vi "Configure Bitfile.vi"(0 "USRP RIO device":T1, 5 "which bitfile":string(combo)="Time", 11 "error in":errorcluster) -> (4 "USRP RIO device":T1, 6 "bitfile":path, 15 "error out":errorcluster)   [LabVIEW 2016]
uses:
  <vilib>/userdefined/Silver/nirio_resource_slv.ctl
  <vilib>/Utility/error.llb/Error Cluster From Error Code.vi
  <vilib>/ErrorRing/Error Ring.xnode
  <vilib>/regexp/Match Regular Expression.xnode
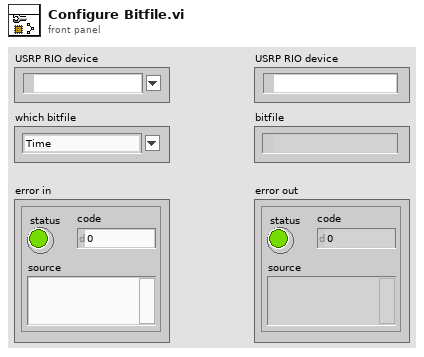
[diagram p1: front panel]
types:
  T1 = typedef "nirio_resource_slv.ctl" = tag
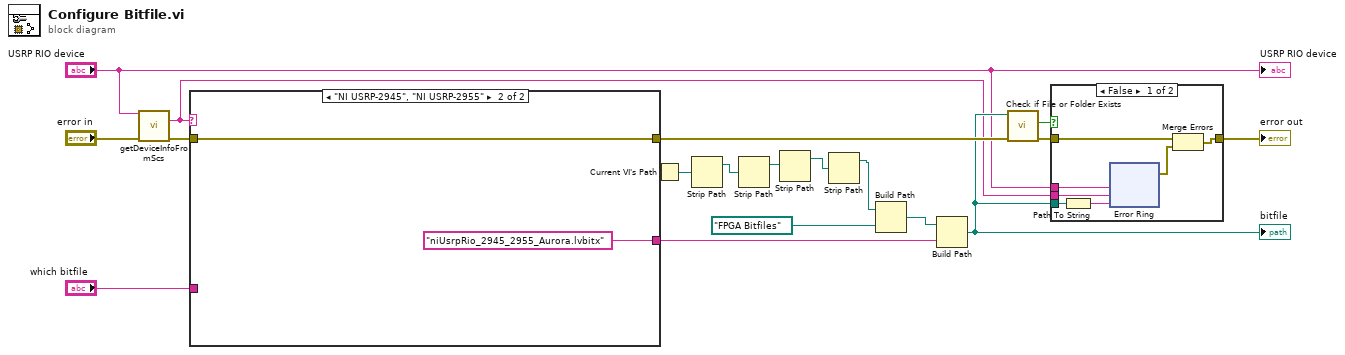
[diagram p0: block diagram]
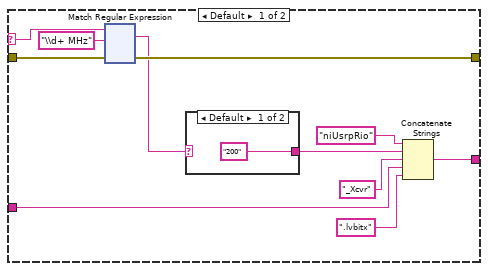
[diagram p3: hidden frame]
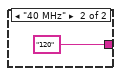
[diagram p4: hidden frame]
diagram:
  n1 = call <vilib>:"getDeviceInfoFromScs.vi"("rio device"="USRP RIO device", "error in"="error in") -> ("product name"=w7:string, "error out"=w11:errorcluster)  [unwired: 9 in, 3 out]
  n2 = case shown="\"NI USRP-2945\", \"NI USRP-2955\"" w7 {
    selector: w7 -> [w19 _]
    tunnel: "which bitfile" -> [w26 _]
    tunnel: w11 -> [w24 w146]
    tunnel: [w23 w146] -> w9
    tunnel: [w20 "niUsrpRio_2945_2955_Aurora.lvbitx" ("f")] -> w10
    frame Default {
      n3 = xnode "Match Regular Expression"("input string"=w19, "regular expression"="\\d+ MHz", "error in"=w24) -> ("whole match"=w22:string, "error out"=w23:errorcluster)  [unwired: 3 in, 3 out]
      n4 = case shown="Default" w22 {
        tunnel: ["200" ("format string") "120" ("format string")] -> w21
        frame Default {
        }
        frame "40 MHz" {
        }
      }
      n5 = Concatenate Strings("niUsrpRio" ("format string"), w21, "_Xcvr" ("format string"), w26, ".lvbitx" ("format string")) -> (w20:string)
    }
    frame "NI USRP-2945", "NI USRP-2955" {
    }
  }
  n6 = Current VI's Path() -> (path=w18:path)
  n7 = Strip Path(path=w18) -> (stripped path=w15:path)  [unwired: 1 out]
  n8 = Strip Path(path=w15) -> (stripped path=w14:path)  [unwired: 1 out]
  n9 = Strip Path(path=w14) -> (stripped path=w2:path)  [unwired: 1 out]
  n10 = Strip Path(path=w2) -> (stripped path=w1:path)  [unwired: 1 out]
  n11 = Build Path(base path=w1, name or relative path=path "FPGA Bitfiles") -> (appended path=w16:path)
  n12 = Build Path(base path=w16, name or relative path=w10) -> (appended path=w8:path)
  "bitfile" <- w8
  n13 = call <vilib>:"Check if File or Folder Exists.vi"("error in (no error)"=w9, "path"=w8) -> ("error out"=w4:errorcluster, "file or folder exists?"=w3:bool)  [unwired: 7 in, 1 out]
  n14 = case shown="False" w3 {
    tunnel: w8 -> [w154 _]
    tunnel: w7 -> [w152 _]
    tunnel: "USRP RIO device" -> [w151 _]
    tunnel: [w149 w164] -> w5
    tunnel: w4 -> [w150 w164]
    frame False {
      n15 = Path To String(path=w154) -> (string=w153:string)
      n16 = xnode "Error Ring"("parameter 0"=w151, "parameter 1"=w152, "parameter 2"=w153) -> ("error out"=w148:errorcluster)
      n17 = Merge Errors(w150, w148) -> (w149:errorcluster)
    }
    frame True {
    }
  }
  "error out" <- w5
  "USRP RIO device" <- "USRP RIO device"
